vi "Process Differential Capture.vi"(0 "Waveform Array":waveform(dbl)[](array[waveform]), 1 "# of Cycles":u16, 5 "Filter Mode":T1(ring), 7 "Idle Offset Voltage":dbl, 9 "Deadspace VppMAX":dbl, 11 "Deadspace LengthMIN":u16, 12 "Points / Aperture(S)":dbl) -> (4 "Waveform Array Out":waveform(dbl)[](array[waveform]), 6 "Waveform is Valid":bool, 8 "Net DC":dbl)   [LabVIEW 2010]
uses:
  <vilib>/Analysis/NI_AALBase.lvlib
panel:
  out "Processed":waveform(dbl)[](graph)
  out "Raw":waveform(dbl)[](graph)
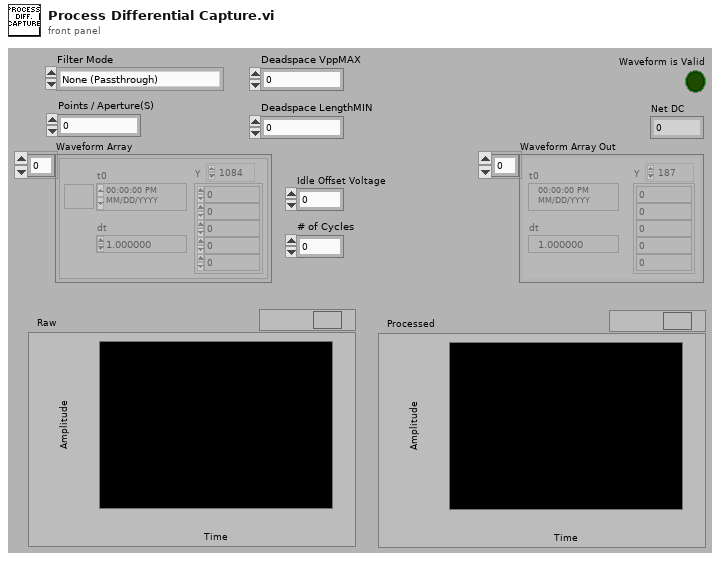
[diagram p1: front panel]
types:
  T1 = enum16{"None (Passthrough)", "Moving Window (Fixed)", "Moving Window (Time)"}
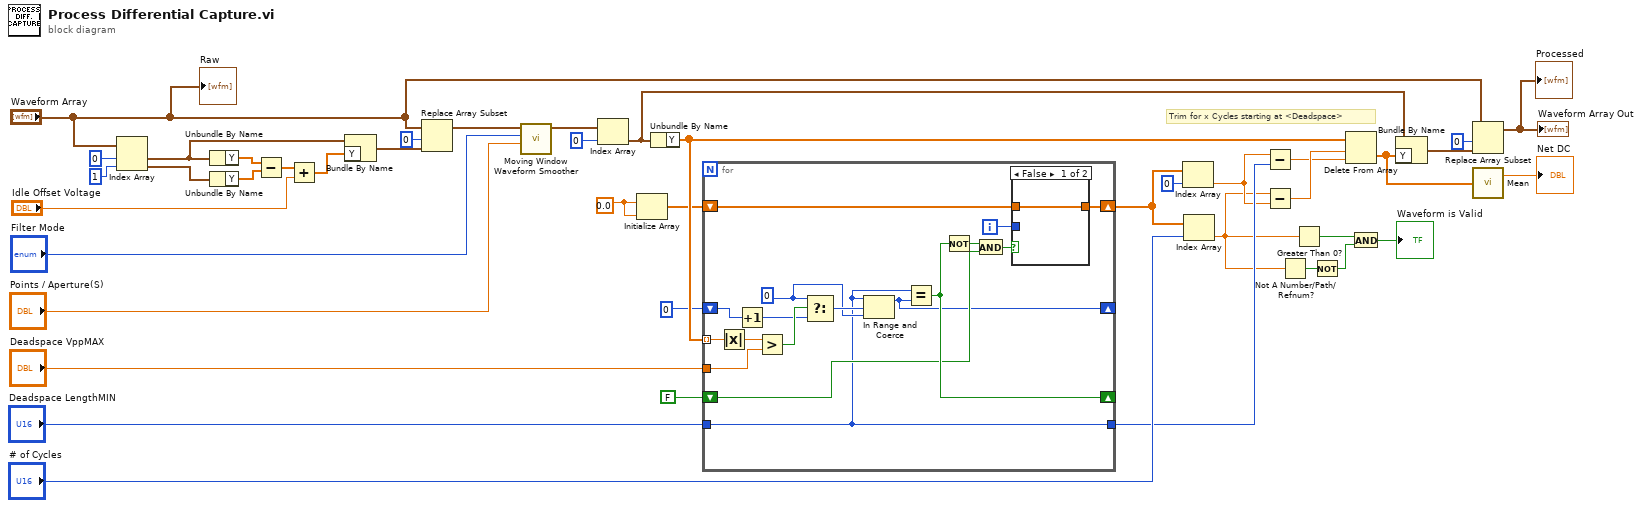
[diagram p0: block diagram]
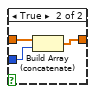
[diagram p2: hidden frame]
diagram:
  w19 = 0.0 ("Deadspace VppMAX")
  # "Trim for x Cycles starting at <Deadspace>"
  n1 = Index Array(array="Waveform Array", index #1=0 ("index"), index #2=1 ("index")) -> (element #1=w34:waveform(dbl), element #2=w40:waveform(dbl))
  n2 = Unbundle By Name(w34) -> ("Y"=w39:dbl[])
  n3 = Unbundle By Name(w40) -> ("Y"=w38:dbl[])
  n4 = Subtract(x=w39, y=w38) -> (x-y=w37:dbl[])
  n5 = Add(x=w37, y="Idle Offset Voltage") -> (x+y=w35:dbl[])
  n6 = Bundle By Name(cluster=w34, "Y"=w35) -> (w33:waveform(dbl))
  n7 = Replace Array Subset(array="Waveform Array", new element=w33, index=0) -> (w31:waveform(dbl)[])
  n8 = call "Moving Window Waveform Smoother.vi"("Points / Aperture(S)"="Points / Aperture(S)", "Filter Mode"="Filter Mode", "Raw Waveforms"=w31) -> ("Filtered Waveforms"=w27:waveform(dbl)[])  [unwired: 8 in]
  n9 = Index Array(array=w27, index=0) -> (element=w24:waveform(dbl))
  n10 = Initialize Array(w19, w19) -> (w20:dbl[])
  n11 = Unbundle By Name(w24) -> ("Y"=w23:dbl[])
  n12 = for {
    tunnel: w23 -> [w57] mode=indexing
    tunnel: "Deadspace VppMAX" -> [w55]
    tunnel: "Deadspace LengthMIN" -> [w45]
    shift-right: [w58] -> w14
    shift-left: w20 -> [w59]
    shift-right: [w49] -> _
    shift-left: FALSE -> [w47]
    shift-right: [w43] -> _
    shift-left: u32 0 ("Deadspace VppMAX") -> [w52]
    tunnel: [w45] -> w11
    i -> [w46]
    w50 = u32 0 ("Deadspace VppMAX")
    n13 = Absolute Value(x=w57) -> (abs(x)=w56:dbl)
    n14 = Increment(x=w52) -> (x+1=w53:u32)
    n15 = Greater?(x=w56, y=w55) -> (0:w54:bool)
    n16 = Select(t=w50, s=w54, f=w53) -> (s? t:f=w51:u32)
    n17 = In Range and Coerce(upper limit=w45, x=w51, lower limit=w50) -> (coerced(x)=w43:u32)  [unwired: 1 out]
    n18 = Equal?(x=w45, y=w43) -> (x = y?=w49:bool)
    n19 = Not(x=w49) -> (.not. x?=w48:bool)
    n20 = And(x=w48, y=w47) -> (x .and. y?=w44:bool)
    n21 = case shown="False" w44 {
      tunnel: w59 -> [w60 w63]
      tunnel: [w60 w62] -> w58
      tunnel: w46 -> [_ w61]
      frame False {
      }
      frame True {
        n22 = Build Array (concatenate)(w63, w61) -> (w62:dbl[])
      }
    }
  }
  n23 = Index Array(array=w14, index=0) -> (element=w10:dbl)
  n24 = Index Array(array=w14, index="# of Cycles") -> (element=w8:dbl)
  n25 = Subtract(x=w10, y=w11) -> (x-y=w12:dbl)
  n26 = Subtract(x=w8, y=w10) -> (x-y=w13:dbl)
  n27 = Not A Number/Path/Refnum?(number/path/refnum=w8) -> (NaN/Path/Refnum?=w9:bool)
  n28 = Greater Than 0?(x=w8) -> (x > 0?=w7:bool)
  n29 = Not(x=w9) -> (.not. x?=w6:bool)
  n30 = Delete From Array(array=w23, length=w13, index=w12) -> (deleted portion=w4:dbl[])  [unwired: 1 out]
  n31 = And(x=w7, y=w6) -> (x .and. y?=→"Waveform is Valid":bool)
  n32 = Bundle By Name(cluster=w24, "Y"=w4) -> (w26:waveform(dbl))
  n33 = Replace Array Subset(array="Waveform Array", new element=w26, index=0) -> (→"Waveform Array Out" →"Processed":waveform(dbl)[])
  n34 = call <vilib>:"Mean.vi"("X"=w4) -> ("mean"=→"Net DC":dbl)  [unwired: 1 out]
  "Raw" <- "Waveform Array"
